vi "Get Microstep Factor.vi"(4 "error in (no error)":errorcluster, 6 "Axis (1)":i32=1 min=1 max=3, 7 "VISA resource name":refnum<visa-resource-name>) -> (0 "error out":errorcluster, 2 "Microstep factor":i32, 3 "VISA resource name out":refnum<visa-resource-name>)   [LabVIEW 2020, in "Newport ESP301.lvlib"]
doc: "Reports the current setting for microstep factor of a Newport Unidrive compatible programmable driver with step motor axis."
uses:
  Newport ESP301.lvlib
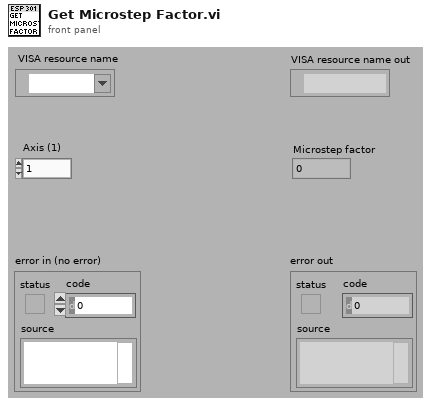
[diagram p1: front panel]
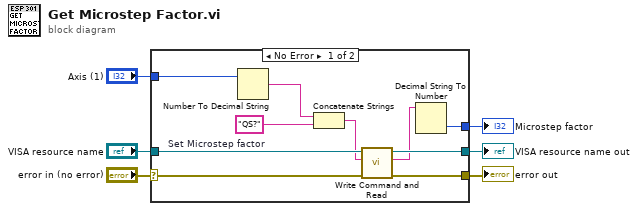
[diagram p0: block diagram]
diagram:
  n1 = case shown="No Error" "error in (no error)" {
    selector: "error in (no error)" -> [w15 w18]
    tunnel: [w8 w18] -> w6
    tunnel: "VISA resource name" -> [w16 w17]
    tunnel: [w10 w17] -> w5
    tunnel: "Axis (1)" -> [w12 _]
    tunnel: [w9 _] -> w1
    frame No Error {
      w13 = "QS?"  # Set Microstep factor
      n2 = Number To Decimal String(number=w12) -> (decimal integer string=w14:string)  [unwired: 1 out]
      n3 = Concatenate Strings(w14, w13) -> (w11:string)
      n4 = call "Write Command and Read.vi"("error in (no error)"=w15, "Command"=w11, "VISA resource name"=w16) -> ("error out"=w8:errorcluster, "Returned string"=w7:string, "VISA resource name out"=w10:refnum<visa-resource-name>)  [unwired: 2 in, 2 out]
      n5 = Decimal String To Number(string=w7) -> (number=w9:i32)  [unwired: 1 in, 2 out]
    }
    frame Error {
    }
  }
  "error out" <- w6
  "VISA resource name out" <- w5
  "Microstep factor" <- w1
